vi "SaveMotorData.vi"(9 "Turret Motor Characteristics":T2, 10 "Drive Motor Characteristics":T2, 11 "Refnum in":T1) -> (3 "Refnum out":T1)   [LabVIEW 2014]
uses:
  <vilib>/Utility/config.llb/Config Data RefNum.ctl
  <vilib>/Utility/config.llb/Write Key (Double).vi
  <vilib>/Utility/config.llb/NI_LVConfig.lvlib
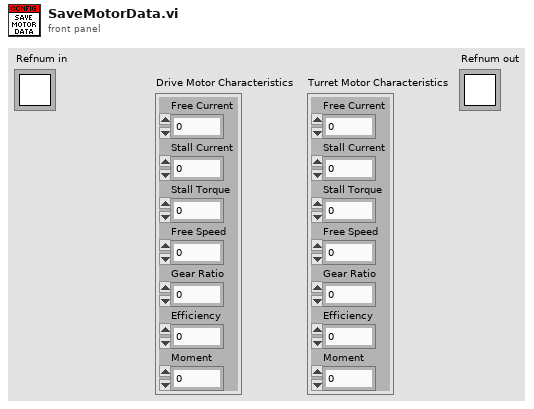
[diagram p1: front panel]
types:
  T1 = typedef "NI_LVConfig.lvlib/Config Data RefNum.ctl" = refnum<k1>
  T2 = cluster{"Free Current":dbl, "Stall Current":dbl, "Stall Torque":dbl, "Free Speed":dbl, "Gear Ratio":dbl, "Efficiency":dbl, "Moment":dbl}
  T3 = cluster{"Free Current":dbl, "Stall Current":dbl, "Stall Torque":dbl, "Free Speed":dbl, "Gear Ratio":dbl, "Efficiency":dbl, "Moment":dbl}[]
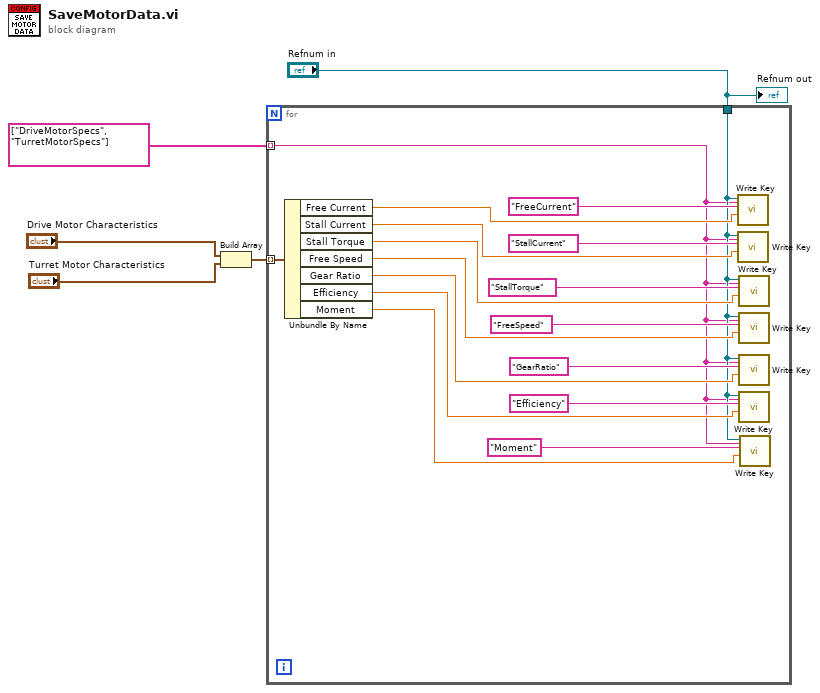
[diagram p0: block diagram]
diagram:
  n1 = Build Array("Drive Motor Characteristics", "Turret Motor Characteristics") -> (w5:T3)
  n2 = for {
    tunnel: w5 -> [w8] mode=indexing
    tunnel: "Refnum in" -> [w7]
    tunnel: string[] ["DriveMotorSpecs", "TurretMotorSpecs"] -> [w6] mode=indexing
    n3 = Unbundle By Name(w8) -> ("Free Current"=w21:dbl, "Stall Current"=w19:dbl, "Stall Torque"=w16:dbl, "Free Speed"=w15:dbl, "Gear Ratio"=w11:dbl, "Efficiency"=w10:dbl, "Moment"=w9:dbl)
    n4 = call-poly <vilib>:"Write Key.vi"("section"=w6, "value"=w21, "key"="FreeCurrent", "refnum"=w7) -> ()  [unwired: 5 in, 3 out]
    n5 = call-poly <vilib>:"Write Key.vi"("section"=w6, "value"=w19, "key"="StallCurrent", "refnum"=w7) -> ()  [unwired: 5 in, 3 out]
    n6 = call-poly <vilib>:"Write Key.vi"("section"=w6, "value"=w16, "key"="StallTorque", "refnum"=w7) -> ()  [unwired: 5 in, 3 out]
    n7 = call-poly <vilib>:"Write Key.vi"("section"=w6, "value"=w15, "key"="FreeSpeed", "refnum"=w7) -> ()  [unwired: 5 in, 3 out]
    n8 = call-poly <vilib>:"Write Key.vi"("section"=w6, "value"=w11, "key"="GearRatio", "refnum"=w7) -> ()  [unwired: 5 in, 3 out]
    n9 = call-poly <vilib>:"Write Key.vi"("section"=w6, "value"=w10, "key"="Efficiency", "refnum"=w7) -> ()  [unwired: 5 in, 3 out]
    n10 = call-poly <vilib>:"Write Key.vi"("section"=w6, "value"=w9, "key"="Moment", "refnum"=w7) -> ()  [unwired: 5 in, 3 out]
  }
  "Refnum out" <- "Refnum in"
